vi "Test_ConstructTransport_NoFormatString_NoError.vi"(8 "error in (no error)":errorcluster, 11 "TestCase in":refnum<class "TestFormattedStringBinding.lvclass">) -> (0 "error out":errorcluster, 3 "TestCase out":refnum<class "TestFormattedStringBinding.lvclass">)   [LabVIEW 2017, in "TestFormattedStringBinding.lvclass"]
uses:
  TestFormattedStringBinding.lvclass
  Source/Concrete/FormattedStringBinding/FormattedStringBinding.lvclass/FormattedStringBinding.ctl
  Source/Concrete/FormattedStringBinding/FormattedStringBinding.lvclass
  C:/Git/composed-transport/Source/Concrete/TerminalValueBinding/TerminalValueBinding.lvclass
  <vilib>/Utility/error.llb/Error Cluster From Error Code.vi
  Source/Concrete/TerminalValueBinding/Construct Terminal Value Binding.vi
panel:
  in  "String":string
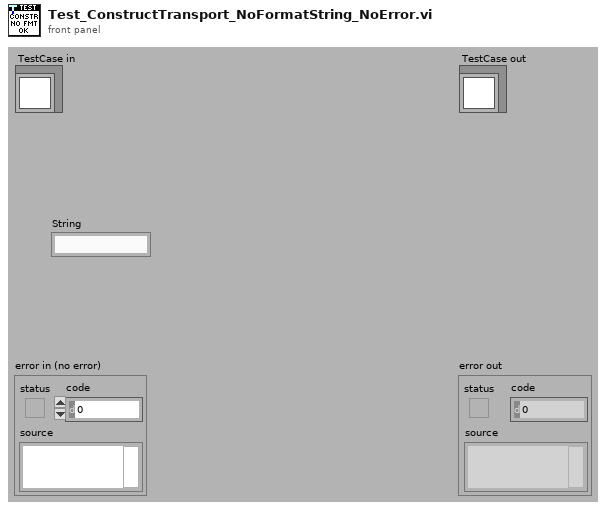
[diagram p1: front panel]
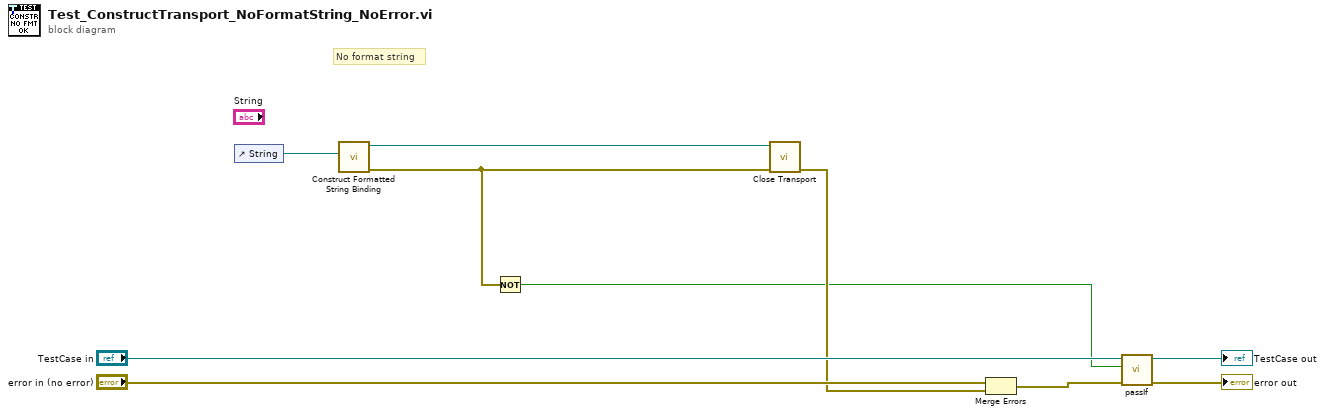
[diagram p0: block diagram]
diagram:
  # "No format string"
  n1 = control-ref of="String"() -> (w5:refnum<vi>)
  n2 = call "Construct Formatted String Binding.vi"("Str Refnum"=w5) -> ("error out"=w1:errorcluster, "FormattedStringBinding"=w3:refnum<class "FormattedStringBinding.lvclass">)  [unwired: 9 in]
  n3 = Not(x=w1) -> (.not. x?=w2:bool)
  n4 = call-dynamic "Close Transport.vi"("error in (no error)"=w1, "ITransport in"=w3) -> ("error out"=w4:errorcluster)  [unwired: 9 in]
  n5 = Merge Errors("error in (no error)", w4) -> (w6:errorcluster)
  n6 = call-dynamic "passIf.vi"("error in (no error)"=w6, "pass"=w2, "TestCase in"="TestCase in") -> ("error out"=→"error out":errorcluster, "TestCase out"=→"TestCase out":refnum<class "TestFormattedStringBinding.lvclass">)  [unwired: 7 in]
